vi "Verify.vi"(8 "error in (no error)":errorcluster, 10 "Comparator":refnum<class "Comparator.lvclass">, 11 "Mock In":refnum<class "Mock.lvclass">) -> (0 "error out":errorcluster, 1 "Errors":errorcluster[](array[cluster]), 2 "Results":cluster{"Passed?":bool, "Message":string}[](array[cluster]))   [LabVIEW 2020, in "Mock.lvclass"]
uses:
  Mock.lvclass
  Comparator/Comparator.lvclass
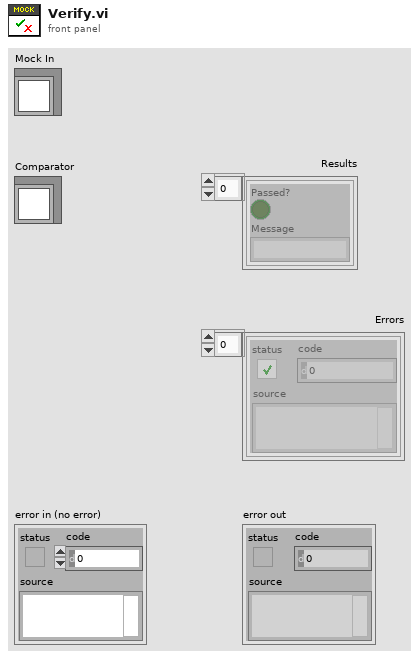
[diagram p1: front panel]
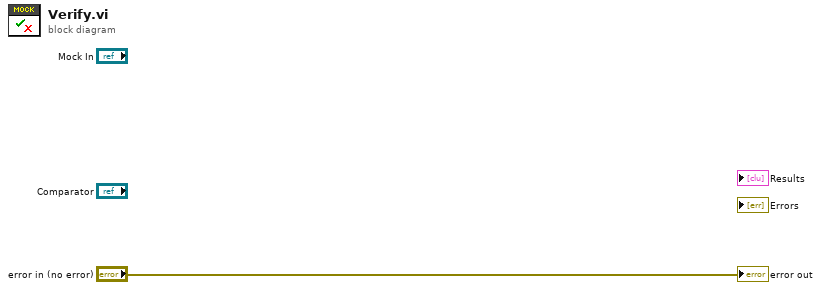
[diagram p0: block diagram]
diagram:
  "error out" <- "error in (no error)"
